vi "Example_2(Hardware).vi"() -> ()   [LabVIEW 2013]
doc: "This VI demonstaits how to write to and read back data from a MIPI device. To run this VI:\n1) Change Resource name to the name of your HSDIO card\n2) The MIPI clock will run at <Sample Clock Rate>/<Oversample Factor>. This is 26 MHz (full rate). If your device should be run at a slower rate, decrease the sample clock rate and (or) increase the oversample rate.\n3. At 104MHz, the RTD value should be ~5 for a 1.5 meter cable. If you are running at a different clock rate or using a different length cable, adjust the RTD Compensation value so the MIPI data is stable at the falling edge of the clock. If you need futher timing adjustment, consider setting the data position to \"Delay from Sample Clock Rising Edge\" and configuring this delay."
uses:
  Ctrls/Configuration.ctl
  Ctrls/ClockDataChannels.ctl
  <instrlib>/niHSDIO/niHSDIO.llb/niHSDIO_ctl Sample Clock Source Values (ComboBox).ctl
  <instrlib>/niHSDIO/niHSDIO.llb/niHSDIO_ctl Voltage Logic Family Values (Ring).ctl
  Ctrls/RegReadWrite.ctl
  <instrlib>/niHSDIO/niHSDIO.llb/niHSDIO Configure Data Voltage Logic Family.vi
  <instrlib>/niHSDIO/niHSDIO.llb/niHSDIO Configure Digital Edge Start Trigger.vi
  <instrlib>/niHSDIO/niHSDIO.llb/niHSDIO Configure Initial State (String).vi
  <instrlib>/niHSDIO/niHSDIO.llb/niHSDIO Configure Idle State (String).vi
  <instrlib>/niHSDIO/niHSDIO.llb/niHSDIO Write Named Waveform (WDT).vi
  <instrlib>/niHSDIO/niHSDIO.llb/niHSDIO Fetch Waveform (WDT).vi
  <vilib>/Waveform/DWDTOps.llb/DWDT Append Digital Signals.vi
panel:
  out "Parity Error":bool
  out "MIPI Data Read from DUT":cluster{"Read Data":u8[]}[](array[cluster])=[{"Read Data"=[1]}] {"Read Data" format="%.0x"}
  in  "Register Read/Write":T1={"Slave Address"=15, "Register"=26, "Data"=1} {"Data" format="%.0b"; "Register" max=31 format="%.0x"; "Slave Address" max=15 format="%.0x"}
  in  "RTD Compensation Value":i32=4 min=0 max=29
  out "Digital Waveform Graph":digitalwaveform(graph)={"t0"=timestamp(3403282811.6192408 s since 1904-01-01), "dt"=9.615384615384615e-09, "Y"={"transitions"=[], "data"=[[1, 0, 1, 0], [1, 0, 1, 0], [1, 0, 1, 0], [1, 0, 1, 0], [1, 0, 1, 0], [1, 0, 1, 0], [1, 0, 1, 0], [0, 0, 1, 0], [0, 0, 0, 0], [0, 0, 0, 0], [0, 0, 0, 0], [0, 0, 0, 0], [0, 0, 0, 0], [0, 0, 0, 0], [0, 0, 0, 0], [1, 1, 0, 0], [1, 1, 1, 1], [1, 1, 1, 1], [1, 1, 1, 1], [1, 0, 1, 1], [1, 0, 1, 0], [1, 0, 1, 0], [1, 0, 1, 0], [1, 1, 1, 0], [1, 1, 1, 1], [1, 1, 1, 1], [1, 1, 1, 1], [1, 0, 1, 1], [1, 0, 1, 0], [1, 0, 1, 0], [1, 0, 1, 0], [1, 1, 1, 0], [1, 1, 1, 1], [1, 1, 1, 1], [1, 1, 1, 1], [1, 0, 1, 1], [1, 0, 1, 0], [1, 0, 1, 0], [1, 0, 1, 0], [1, 1, 1, 0], [1, 1, 1, 1], [1, 1, 1, 1], [1, 1, 1, 1], [1, 0, 1, 1], [1, 0, 1, 0], [1, 0, 1, 0], [1, 0, 1, 0], [0, 1, 1, 0], [0, 1, 0, 1], [0, 1, 0, 1], [0, 1, 0, 1], [0, 0, 0, 1], [0, 0, 0, 0], [0, 0, 0, 0], [0, 0, 0, 0], [1, 1, 0, 0], [1, 1, 1, 1], [1, 1, 1, 1], [1, 1, 1, 1], [1, 0, 1, 1], [1, 0, 1, 0], [1, 0, 1, 0], [1, 0, 1, 0], [0, 1, 1, 0], [0, 1, 0, 1], [0, 1, 0, 1], [0, 1, 0, 1], [0, 0, 0, 1], [0, 0, 0, 0], [0, 0, 0, 0], [0, 0, 0, 0], [1, 1, 0, 0], [1, 1, 1, 1], [1, 1, 1, 1], [1, 1, 1, 1], [1, 0, 1, 1], [1, 0, 1, 0], [1, 0, 1, 0], [1, 0, 1, 0], [1, 1, 1, 0], [1, 1, 1, 1], [1, 1, 1, 1], [1, 1, 1, 1], [1, 0, 1, 1], [1, 0, 1, 0], [1, 0, 1, 0], [1, 0, 1, 0], [0, 1, 1, 0], [0, 1, 0, 1], [0, 1, 0, 1], [0, 1, 0, 1], [0, 0, 0, 1], [0, 0, 0, 0], [0, 0, 0, 0], [0, 0, 0, 0], [1, 1, 0, 0], [1, 1, 1, 1], [1, 1, 1, 1], [1, 1, 1, 1], [1, 0, 1, 1], [1, 0, 1, 0], [1, 0, 1, 0], [1, 0, 1, 0], [0, 1, 1, 0], [0, 1, 0, 1], [0, 1, 0, 1], [0, 1, 0, 1], [0, 0, 0, 1], [0, 0, 0, 0], [0, 0, 0, 0], [0, 0, 0, 0], [1, 1, 0, 0], [1, 1, 1, 1], [1, 1, 1, 1], [1, 1, 1, 1], [1, 0, 1, 1], [1, 0, 1, 0], [1, 0, 1, 0], [1, 0, 1, 0], [0, 1, 1, 0], [0, 1, 0, 1], [0, 1, 0, 1], [0, 1, 0, 1], [0, 0, 0, 1], [0, 0, 0, 0], [0, 0, 0, 0], [0, 0, 0, 0], [0, 1, 0, 0], [0, 1, 0, 1], [0, 1, 0, 1], [0, 1, 0, 1], [0, 0, 0, 1], [0, 0, 0, 0], [0, 0, 0, 0], [0, 0, 0, 0], [0, 1, 0, 0], [0, 1, 0, 1], [0, 1, 0, 1], [0, 1, 0, 1], [0, 0, 0, 1], [0, 0, 0, 0], [0, 0, 0, 0], [0, 0, 0, 0], [0, 1, 0, 0], [0, 1, 0, 1], [0, 1, 0, 1], [0, 1, 0, 1], [0, 0, 0, 1], [0, 0, 0, 0], [0, 0, 0, 0], [0, 0, 0, 0], [0, 1, 0, 0], [0, 1, 0, 1], [0, 1, 0, 1], [0, 1, 0, 1], [0, 0, 0, 1], [0, 0, 0, 0], [0, 0, 0, 0], [0, 0, 0, 0], [0, 1, 0, 0], [0, 1, 0, 1], [0, 1, 0, 1], [0, 1, 0, 1], [0, 0, 0, 1], [0, 0, 0, 0], [0, 0, 0, 0], [0, 0, 0, 0], [0, 1, 0, 0], [0, 1, 0, 1], [0, 1, 0, 1], [0, 1, 0, 1], [0, 0, 0, 1], [0, 0, 0, 0], [0, 0, 0, 0], [0, 0, 0, 0], [1, 1, 0, 0], [1, 1, 1, 1], [1, 1, 1, 1], [1, 1, 1, 1], [1, 0, 1, 1], [1, 0, 1, 0], [1, 0, 1, 0], [1, 0, 1, 0], [0, 1, 1, 0], [0, 1, 0, 1], [0, 1, 0, 1], [0, 1, 0, 1], [0, 0, 0, 1], [0, 0, 0, 0], [0, 0, 0, 0], [0, 0, 0, 0], [0, 1, 0, 0], [0, 1, 0, 1], [0, 1, 0, 1], [0, 1, 0, 1], [0, 0, 0, 1], [0, 0, 0, 0], [0, 0, 0, 0], [0, 0, 0, 0], [1, 0, 0, 0], [1, 0, 1, 0], [1, 0, 1, 0], [1, 0, 1, 0], [1, 0, 1, 0], [1, 0, 1, 0], [1, 0, 1, 0], [1, 0, 1, 0], [0, 0, 1, 0], [0, 0, 0, 0], [0, 0, 0, 0], [0, 0, 0, 0], [0, 0, 0, 0], [0, 0, 0, 0], [0, 0, 0, 0], [0, 0, 0, 0], [1, 1, 0, 0], [1, 1, 1, 1], [1, 1, 1, 1], [1, 1, 1, 1], [1, 0, 1, 1], [1, 0, 1, 0], [1, 0, 1, 0], [1, 0, 1, 0], [1, 1, 1, 0], [1, 1, 1, 1], [1, 1, 1, 1], [1, 1, 1, 1], [1, 0, 1, 1], [1, 0, 1, 0], [1, 0, 1, 0], [1, 0, 1, 0], [1, 1, 1, 0], [1, 1, 1, 1], [1, 1, 1, 1], [1, 1, 1, 1], [1, 0, 1, 1], [1, 0, 1, 0], [1, 0, 1, 0], [1, 0, 1, 0], [1, 1, 1, 0], [1, 1, 1, 1], [1, 1, 1, 1], [1, 1, 1, 1], [1, 0, 1, 1], [1, 0, 1, 0], [1, 0, 1, 0], [1, 0, 1, 0], [0, 1, 1, 0], [0, 1, 0, 1], [0, 1, 0, 1], [0, 1, 0, 1], [0, 0, 0, 1], [0, 0, 0, 0], [0, 0, 0, 0], [0, 0, 0, 0], [1, 1, 0, 0], [1, 1, 1, 1], [1, 1, 1, 1], [1, 1, 1, 1], [1, 0, 1, 1], [1, 0, 1, 0], [1, 0, 1, 0], [1, 0, 1, 0], [1, 1, 1, 0], [1, 1, 1, 1], [1, 1, 1, 1], [1, 1, 1, 1], [1, 0, 1, 1], [1, 0, 1, 0], [1, 0, 1, 0], [1, 0, 1, 0], [1, 1, 1, 0], [1, 1, 1, 1], [1, 1, 1, 1], [1, 1, 1, 1], [1, 0, 1, 1], [1, 0, 1, 0], [1, 0, 1, 0], [1, 0, 1, 0], [1, 1, 1, 0], [1, 1, 1, 1], [1, 1, 1, 1], [1, 1, 1, 1], [1, 0, 1, 1], [1, 0, 1, 0], [1, 0, 1, 0], [1, 0, 1, 0], [0, 1, 1, 0], [0, 1, 0, 1], [0, 1, 0, 1], [0, 1, 0, 1], [0, 0, 0, 1], [0, 0, 0, 0], [0, 0, 0, 0], [0, 0, 0, 0], [1, 1, 0, 0], [1, 1, 1, 1], [1, 1, 1, 1], [1, 1, 1, 1], [1, 0, 1, 1], [1, 0, 1, 0], [1, 0, 1, 0], [1, 0, 1, 0], [0, 1, 1, 0], [0, 1, 0, 1], [0, 1, 0, 1], [0, 1, 0, 1], [0, 0, 0, 1], [0, 0, 0, 0], [0, 0, 0, 0], [0, 0, 0, 0], [0, 1, 0, 0], [0, 1, 0, 1], [0, 1, 0, 1], [0, 1, 0, 1], [0, 0, 0, 1], [0, 0, 0, 0], [0, 0, 0, 0], [0, 0, 0, 0], [0, 1, 0, 0], [0, 1, 0, 1], [0, 1, 0, 1], [0, 1, 0, 1], [0, 0, 0, 1], [0, 0, 0, 0], [0, 0, 0, 0], [0, 0, 0, 0], [0, 1, 0, 0], [0, 1, 5, 1], [0, 1, 5, 1], [0, 1, 5, 1], [0, 0, 5, 1], [0, 0, 4, 0], [0, 0, 5, 0], [0, 0, 5, 0], [0, 1, 5, 0], [0, 1, 5, 1], [0, 1, 5, 1], [0, 1, 5, 1], [0, 0, 5, 1], [0, 0, 3, 0], [0, 0, 5, 0], [0, 0, 5, 0], [0, 1, 5, 0], [0, 1, 5, 1], [0, 1, 5, 1], [0, 1, 5, 1], [0, 0, 5, 1], [0, 0, 4, 0], [0, 0, 5, 0], [0, 0, 5, 0], [0, 1, 5, 0], [0, 1, 5, 1], [0, 1, 5, 1], [0, 1, 5, 1], [0, 0, 5, 1], [0, 0, 3, 0], [0, 0, 5, 0], [0, 0, 5, 0], [0, 1, 5, 0], [0, 1, 5, 1], [0, 1, 5, 1], [0, 1, 5, 1], [0, 0, 5, 1], [0, 0, 4, 0], [0, 0, 5, 0], [0, 0, 5, 0], [0, 1, 5, 0], [0, 1, 5, 1], [0, 1, 5, 1], [0, 1, 5, 1], [0, 0, 5, 1], [0, 0, 3, 0], [0, 0, 5, 0], [0, 0, 5, 0], [0, 1, 5, 0], [0, 1, 5, 1], [0, 1, 5, 1], [0, 1, 5, 1], [0, 0, 5, 1], [0, 0, 4, 0], [0, 0, 5, 0], [0, 0, 5, 0], [0, 1, 5, 0], [0, 1, 5, 1], [0, 1, 5, 1], [1, 1, 5, 1], [1, 0, 5, 1], [1, 0, 3, 0], [1, 0, 5, 0], [1, 0, 5, 0], [1, 1, 5, 0], [1, 1, 5, 1], [1, 1, 5, 1], [0, 1, 5, 1], [0, 0, 5, 1], [0, 0, 4, 0], [1, 0, 5, 0], [0, 0, 5, 0], [0, 1, 5, 0], [0, 1, 0, 1], [0, 1, 0, 1], [0, 1, 0, 1], [0, 0, 0, 1], [0, 0, 0, 0], [0, 0, 0, 0], [0, 0, 0, 0], [0, 0, 0, 0]]}}
  in  "Configuratation":T2={"Samples to Allocate"=10000, "Oversample Factor"=4, "Clock Channel"=enum."0", "Data Channel"=enum."1"} {"Oversample Factor" min=1 max=254; "Samples to Allocate" min=1}
  out "Number of Sample Errors Read":i32=6
  in  "Sample Clock Rate":dbl=104000000.0 format="%#_6p"
  in  "Resource name":refnum<k15>="PXI1Slot4"
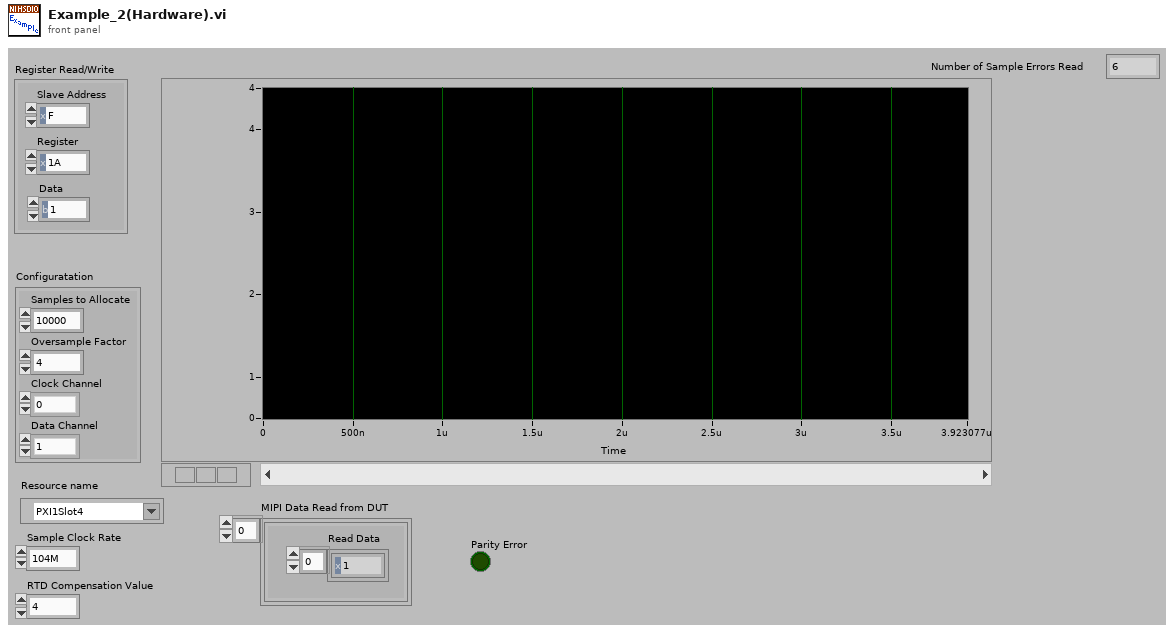
[diagram p1: front panel]
types:
  T1 = cluster{"Slave Address":u8, "Register":u8, "Data":u8}
  T2 = typedef "Configuration.ctl" = cluster{"Samples to Allocate":i32, "Oversample Factor":u8, "Clock Channel":T3, "Data Channel":T3}
  T3 = typedef "ClockDataChannels.ctl" = enum16{"0", "1"}
  T4 = typedef "RegReadWrite.ctl" = cluster{"Slave Address":u8, "Register":u8, "Data":u8}
  T5 = typedef "niHSDIO_ctl Voltage Logic Family Values (Ring).ctl" = i32
  T6 = typedef "niHSDIO_ctl Sample Clock Source Values (ComboBox).ctl" = string
  T7 = typedef "RFFE_Data.ctl" = cluster{"Clock Channel":T3, "Data Channel":T3, "Oversample Factor":u8, "Zero Array":u8[], "One Array":u8[], "Z Array ":u8[], "H Array":u8[], "L Array":u8[], "X Array":u8[], "Toggle (high to low)":u8[]}
  T8 = typedef "ReadInfo.ctl" = cluster{"Expected Value(s)":u8[], "Compare Locations":u32[]}
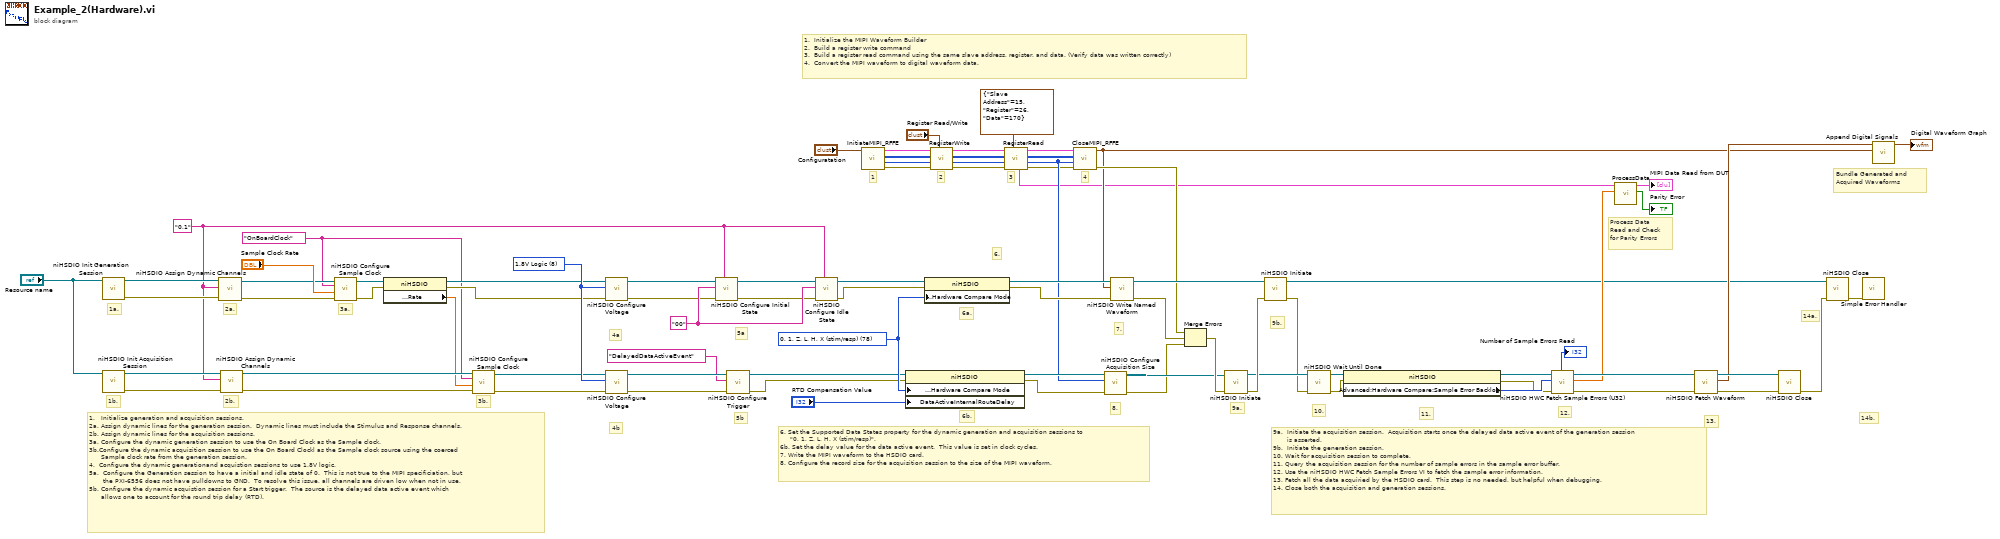
[diagram p0: block diagram]
diagram:
  w10 = "00" ("idle state")
  w3 = "0,1" ("channel list (all:\"\")")
  w48 = T5 8 items=["5.0V Logic"=5, "3.3V Logic"=6, "2.5V Logic"=7, "1.8V Logic"=8, "1.5V Logic"=80, "1.2V Logic"=81] ("logic family (3.3V logic)")
  w66 = 78 items=["0, 1 (binary)"=77, "0, 1, Z (tristate)"=83, "0, 1, Z, L, H, X (stim/resp)"=78, "L, H, X (resp only)"=79] ("Advanced:Supported Data States")
  w31 = T6 "OnBoardClock" ("clock source (on board clock)")
  # "4"
  # "3"
  # "2"
  # "1"
  # "1.  Initialize the MIPI Waveform Builder\n2.  Build a register write command\n3.  Build a register read command using the same slave address, register, and data. (Verify data was written correctly)\n4.  Convert the MIPI waveform to digital waveform data."
  # "Bundle Generated and Acquired Waveforms"
  # "5a"
  # "Process Data Read and Check for Parity Errors"
  # "4b"
  # "4a"
  # "13."
  # "6. Set the Supported Data States property for the dynamic generation and acquisition sessions to \n     \"0, 1, Z, L, H, X (stim/resp)\".\n6b. Set the delay value for the data active event.  This value is set in clock cycles.\n7. Write the MIPI waveform to the HSDIO card.\n8. Configure the record size for the acquisition session to the size of the MIPI waveform."
  # "6."
  # "1.   Initialize generation and acquisition sessions.\n2a. Assign dynamic lines for the generation session.  Dynamic lines must include the Stimulus and Response channels.\n2b. Assign dynamic lines for the acquisition sessions.\n3a. Configure the dynamic generation session to use the On Board Clock as the Sample clock.\n3b.Configure the dynamic acquisition session to use the On Board Clockl as the Sample clock source using the coerced \n      Sample clock rate from the generation session.\n4.  Configure the dynamic generationand acquistion sessions to use 1.8V logic.\n5a.  Configure the Generation session to have a initial and idle state of 0.  This is not true to the MIPI specificiation, but\n       the PXI-6556 does not have pulldowns to GND.  To resolve this issue, all channels are driven low when not in use.\n5b. Configure the dynamic acquistion session for a Start trigger.  The source is the delayed data active event which\n      allows one to account for the round trip delay (RTD)."
  # "14b."
  # "12."
  # "11."
  # "10."
  # "9b."
  # "9a."
  # "9a.  Initiate the acquisition session.  Acquisition starts once the delayed data active event of the generation session\n       is asserted. \n9b.  Initiate the generation session.\n10. Wait for acquisition session to complete.\n11. Query the acquisition session for the number of sample errors in the sample error buffer.\n12. Use the niHSDIO HWC Fetch Sample Errors VI to fetch the sample error information.\n13. Fetch all the data acquiried by the HSDIO card.  This step is no needed, but helpful when debugging.\n14. Close both the acquisition and generation sessions."
  # "8."
  # "7."
  # "6b."
  # "6a."
  # "5b"
  # "3b."
  # "3a."
  # "2b."
  # "2a."
  # "1b."
  # "1a."
  # "14a."
  n1 = call <instrlib>:"niHSDIO Init Generation Session.vi"("resource name"="Resource name") -> ("error out"=w34:errorcluster, "instrument handle out"=w35:refnum<k15>)  [unwired: 9 in]
  n2 = call <instrlib>:"niHSDIO Init Acquisition Session.vi"("resource name"="Resource name") -> ("error out"=w38:errorcluster, "instrument handle out"=w77:refnum<k15>)  [unwired: 9 in]
  n3 = call <instrlib>:"niHSDIO Assign Dynamic Channels.vi"("error in (no error)"=w34, "channel list (all:\"\")"=w3, "instrument handle"=w35) -> ("error out"=w64:errorcluster, "instrument handle out"=w65:refnum<k15>)  [unwired: 7 in]
  n4 = call <instrlib>:"niHSDIO Assign Dynamic Channels.vi"("error in (no error)"=w38, "channel list (all:\"\")"=w3, "instrument handle"=w77) -> ("error out"=w56:errorcluster, "instrument handle out"=w57:refnum<k15>)  [unwired: 7 in]
  n5 = call <instrlib>:"niHSDIO Configure Sample Clock.vi"("error in (no error)"=w64, "clock rate (50MHz)"="Sample Clock Rate", "clock source (on board clock)"=w31, "instrument handle"=w65) -> ("error out"=w32:errorcluster, "instrument handle out"=w33:refnum<k15>)  [unwired: 6 in]
  n6 = property on="Property Node" class="niHSDIO"(reference=w33, error in=w32) -> (reference out=w46:refnum<k15>, error out=w47:errorcluster, "Timing:Sample Clock:Rate"=w53:dbl)
  n7 = call <instrlib>:"niHSDIO Configure Sample Clock.vi"("error in (no error)"=w56, "clock rate (50MHz)"=w53, "clock source (on board clock)"=w31, "instrument handle"=w57) -> ("error out"=w30:errorcluster, "instrument handle out"=w29:refnum<k15>)  [unwired: 6 in]
  n8 = call-poly <instrlib>:"niHSDIO Configure Voltage.vi"("error in (no error)"=w47, "logic family (3.3V logic)"=w48, "instrument handle"=w46) -> ("error out"=w6:errorcluster, "instrument handle out"=w7:refnum<k15>)  [unwired: 7 in]
  n9 = call-poly <instrlib>:"niHSDIO Configure Voltage.vi"("error in (no error)"=w30, "logic family (3.3V logic)"=w48, "instrument handle"=w29) -> ("error out"=w27:errorcluster, "instrument handle out"=w28:refnum<k15>)  [unwired: 7 in]
  n10 = call-poly <instrlib>:"niHSDIO Configure Initial State.vi"("channel list"=w3, "error in (no error)"=w6, "initial state"=w10, "instrument handle"=w7) -> ("error out"=w9:errorcluster, "instrument handle out"=w8:refnum<k15>)  [unwired: 6 in]
  n11 = call-poly <instrlib>:"niHSDIO Configure Trigger.vi"("error in (no error)"=w27, "source (PFI 0)"="DelayedDataActiveEvent" ("channel list (all:\"\")"), "instrument handle"=w28) -> ("error out"=w23:errorcluster, "instrument handle out"=w26:refnum<k15>)  [unwired: 7 in]
  n12 = call-poly <instrlib>:"niHSDIO Configure Idle State.vi"("channel list"=w3, "error in (no error)"=w9, "idle state"=w10, "instrument handle"=w8) -> ("error out"=w5:errorcluster, "instrument handle out"=w4:refnum<k15>)  [unwired: 6 in]
  n13 = call "InitiateMIPI_RFFE.vi"("Configuratation In"="Configuratation") -> ("error out"=w45:errorcluster, "Number of Samples Out"=w44:i32, "Data Array"=w43:u8[][], "RFFE_Data"=w41:T7)  [unwired: 7 in]
  n14 = property on="Property Node" class="niHSDIO"(reference=w26, error in=w23, "Advanced:Hardware Compare:Hardware Compare Mode"=w66, "DataActiveInternalRouteDelay"="RTD Compensation Value") -> (reference out=w61:refnum<k15>, error out=w60:errorcluster)
  n15 = property on="Property Node" class="niHSDIO"(reference=w4, error in=w5, "Advanced:Hardware Compare:Hardware Compare Mode"=w66) -> (reference out=w63:refnum<k15>, error out=w62:errorcluster)
  n16 = call "RegisterWrite.vi"("Write Data"="Register Read/Write", "error in (no error)"=w45, "Number of Samples In"=w44, "Data Array"=w43, "RFFE_Data"=w41) -> ("error out"=w21:errorcluster, "Number of Samples Out"=w19:i32, "Data Array Out"=w20:u8[][], "Configuratation Out"=w18:T7)  [unwired: 3 in]
  n17 = call "RegisterRead.vi"("Register Read/Write"=T4 {"Slave Address"=15, "Register"=26, "Data"=170}, "error in (no error)"=w21, "Number of Samples In"=w19, "Data Array"=w20, "RFFE_Data In"=w18) -> ("error out"=w14:errorcluster, "Number of Samples Out out"=w15:i32, "Data Array Out"=w16:u8[][], "RFFE_Data Out"=w17:T7, "Compare Bits Out"=w13:T8[])  [unwired: 2 in]
  n18 = call "CloseMIPI_RFFE.vi"("error in (no error)"=w14, "Number of Samples"=w15, "Data Array"=w16, "RFFE_Data"=w17) -> ("error out"=w49:errorcluster, "Digital Waveform"=w22:digitalwaveform)  [unwired: 6 in]
  n19 = call <instrlib>:"niHSDIO Configure Acquisition Size.vi"("error in (no error)"=w60, "samples per record (1000 samples)"=w15, "instrument handle"=w61) -> ("error out"=w55:errorcluster, "instrument handle out"=w59:refnum<k15>)  [unwired: 7 in]
  n20 = call-poly <instrlib>:"niHSDIO Write Named Waveform.vi"("error in (no error)"=w62, "data"=w22, "instrument handle"=w63) -> ("error out"=w54:errorcluster, "instrument handle out"=w68:refnum<k15>)  [unwired: 7 in]
  n21 = Merge Errors(w49, w54, w55) -> (w67:errorcluster)
  n22 = call <instrlib>:"niHSDIO Initiate.vi"("error in (no error)"=w67, "instrument handle"=w59) -> ("error out"=w76:errorcluster, "instrument handle out"=w74:refnum<k15>)  [unwired: 8 in]
  n23 = call <instrlib>:"niHSDIO Initiate.vi"("error in (no error)"=w76, "instrument handle"=w68) -> ("error out"=w72:errorcluster, "instrument handle out"=w36:refnum<k15>)  [unwired: 8 in]
  n24 = call <instrlib>:"niHSDIO Wait Until Done.vi"("error in (no error)"=w72, "instrument handle"=w74) -> ("error out"=w71:errorcluster, "instrument handle out"=w73:refnum<k15>)  [unwired: 8 in]
  n25 = property on="Property Node" class="niHSDIO"(reference=w73, error in=w71) -> (reference out=w70:refnum<k15>, error out=w69:errorcluster, "Advanced:Hardware Compare:Sample Error Backlog"=w78:i32)
  n26 = call <instrlib>:"niHSDIO HWC Fetch Sample Errors (U32).vi"("error in (no error)"=w69, "sample errors  to read"=w78, "instrument handle"=w70) -> ("error out"=w52:errorcluster, "sample numbers"=w39:dbl[], "instrument handle out"=w51:refnum<k15>, "number of sample errors read"=→"Number of Sample Errors Read":i32)  [unwired: 3 in, 2 out]
  n27 = call "ProcessData.vi"("Error Loacations"=w39, "Read Info"=w13) -> ("Parity Error"=→"Parity Error":bool, "Read MIPI Data"=→"MIPI Data Read from DUT":cluster{"Read Data":u8[]}[])  [unwired: 8 in]
  n28 = call-poly <instrlib>:"niHSDIO Fetch Waveform.vi"("error in (no error)"=w52, "instrument handle"=w51) -> ("error out"=w37:errorcluster, "data"=w42:digitalwaveform, "instrument handle out"=w81:refnum<k15>)  [unwired: 6 in, 1 out]
  n29 = call <instrlib>:"niHSDIO Close.vi"("error in (no error)"=w37, "instrument handle"=w81) -> ("error out"=w82:errorcluster)  [unwired: 9 in]
  n30 = call <instrlib>:"niHSDIO Close.vi"("error in (no error)"=w82, "instrument handle"=w36) -> ("error out"=w80:errorcluster)  [unwired: 9 in]
  n31 = call <vilib>:"Simple Error Handler.vi"("error in (no error)"=w80) -> ()  [unwired: 4 in, 5 out]
  n32 = call-poly <vilib>:"Append Digital Signals.vi"("digital waveform (low bits)"=w22, "digital waveform (high bits)"=w42) -> ("digital waveform out"=→"Digital Waveform Graph":digitalwaveform)  [unwired: 8 in, 1 out]
